vi "Read P T.vi"(1 "correção NTC":dbl, 7 "correçao termopar":dbl) -> (0 "String":string, 2 "Sievert01":dbl, 3 "mean H2 sensor":dbl format="%#_4p", 4 "String 2":string, 5 "mean value T":dbl, 6 "mean value P":dbl, 9 "T Set 1 Output":dbl format="%.4g", 10 "P Set 1 Output 2":dbl format="%.3g", 11 "T Set 2 Output":dbl format="%.4g", 12 "termopar K":dbl format="%.3g", 14 "output NTC":dbl, 15 "P Set 2 Output 2":dbl format="%.3g")   [LabVIEW 2011]
uses:
  <vilib>/Analysis/3filter.llb/Filter Passband Type.ctl
  <vilib>/DAQmx/read.llb/DAQmx Read (Analog 1D DBL 1Chan NSamp).vi
  <vilib>/DAQmx/create/channels.llb/DAQmx Create Channel (AI-Voltage-Basic).vi
  <vilib>/DAQmx/configure/timing.llb/DAQmx Timing (Sample Clock).vi
  <vilib>/DAQmx/miscellaneous.llb/DAQmx Fill In Error Info.vi
  <vilib>/Analysis/3filter.llb/Butterworth Filter (DBL).vi
  <vilib>/Analysis/baseanly.llb/Unimode.vi
  <vilib>/Analysis/5stat.llb/RMS (DBL).vi
  <vilib>/DAQmx/create/channels.llb/DAQmx Create Channel (AI-Temperature-Thermocouple).vi
  <vilib>/Analysis/NI_AALBase.lvlib
  Program Files/National Instruments/LabVIEW 2011/resource/objmgr/daqmx.rc
  <vilib>/gmath/NI_Gmath.lvlib
  <vilib>/Analysis/NI_AALPro.lvlib
panel:
  out "error 4":dbl
  in  "filter type 4":T1
  in  "high cutoff freq: fh 4":dbl=0.45000000000000007 format="%0.2f"
  in  "low cutoff freq: fl 4":dbl=0.12500000000000006 format="%0.4f"
  in  "order 4":i32=2
  in  "intervals 4":i32=20
  out "Rt":dbl
  in  "intervals 3":i32=20
  in  "Statistic 3":T2(ring)
  out "P Set 1 Output 3":dbl format="%.3g"
  out "?":T3(graph)
  out "Data Set 6":dbl[](graph)
  out "?":T3(graph)
  out "Data Set 5":dbl[](graph)
  out "error 3":dbl
  in  "filter type 3":T1
  in  "high cutoff freq: fh 3":dbl=0.45000000000000007 format="%0.2f"
  in  "low cutoff freq: fl 3":dbl=0.12500000000000006 format="%0.4f"
  in  "order 3":i32=2
  out "mean value P 2":dbl
  out "String 3":string
  in  "intervals 2":i32=20
  in  "Statistic 2":T2(ring)
  out "?":T3(graph)
  out "Data Set 4":dbl[](graph)
  out "?":T3(graph)
  out "Data Set 3":dbl[](graph)
  out "error 2":dbl
  in  "filter type 2":T1
  in  "high cutoff freq: fh 2":dbl=0.45000000000000007 format="%0.2f"
  in  "low cutoff freq: fl 2":dbl=0.12500000000000006 format="%0.4f"
  in  "order 2":i32=2
  in  "intervals":i32=20
  in  "Statistic":T2(ring)
  out "?":T3(graph)
  out "Data Set 1":dbl[](graph)
  out "?":T3(graph)
  out "Data Set 2":dbl[](graph)
  out "error":dbl
  in  "filter type":T1
  in  "high cutoff freq: fh":dbl=0.45000000000000007 format="%0.2f"
  in  "low cutoff freq: fl":dbl=0.12500000000000006 format="%0.4f"
  in  "order":i32=2
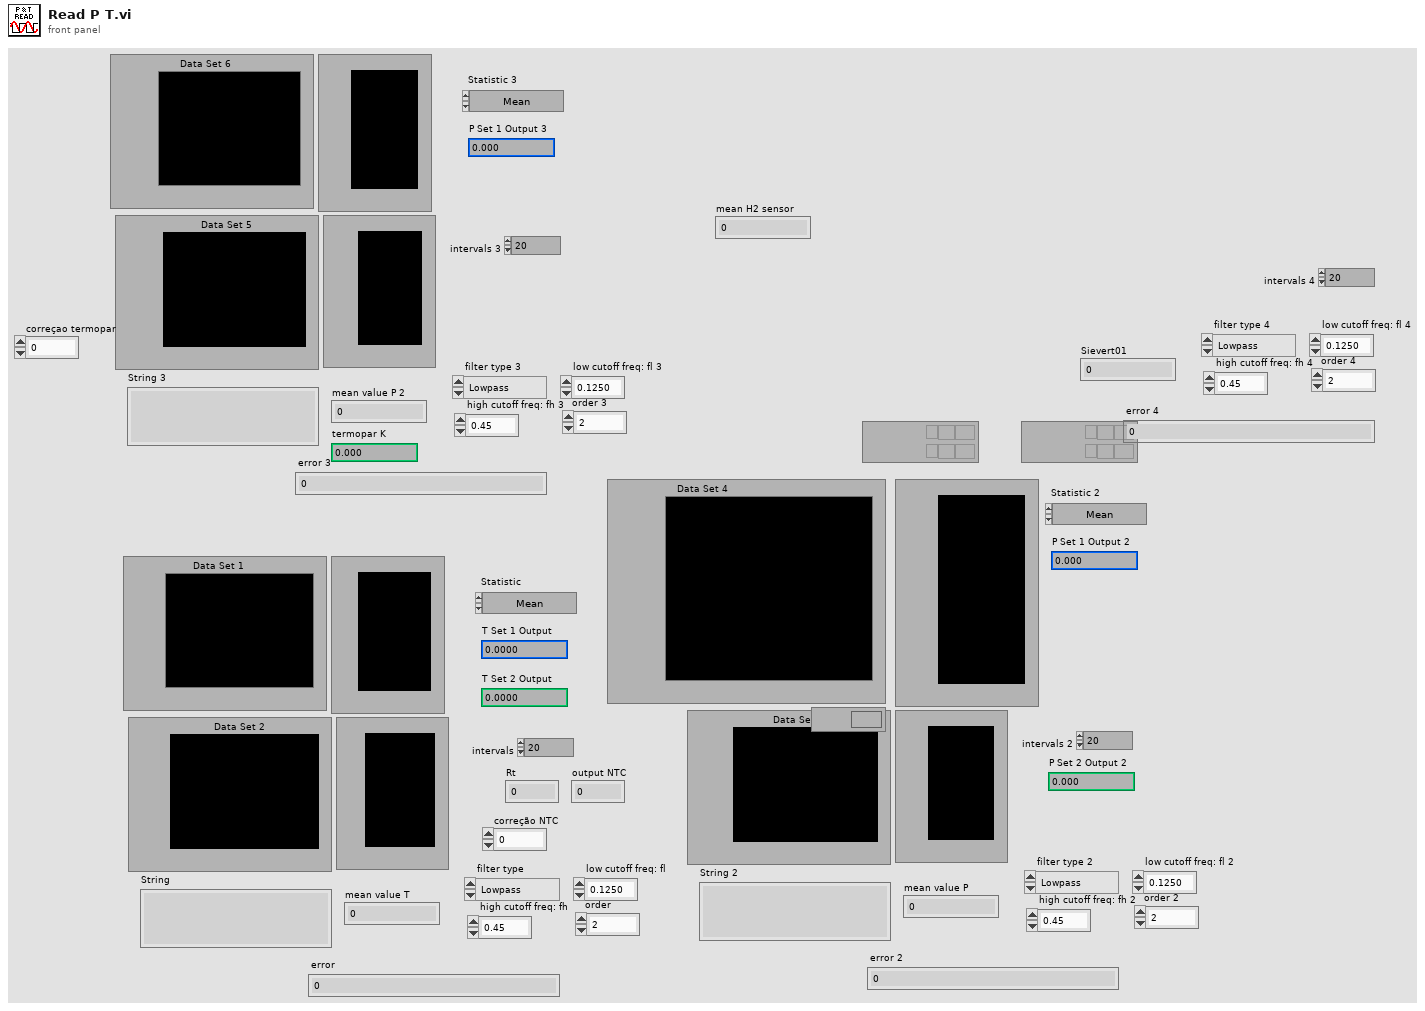
[diagram p1: front panel]
types:
  T1 = typedef "NI_AALBase.lvlib/Filter Passband Type.ctl" = enum32{"Lowpass", "Highpass", "Bandpass", "Bandstop"}
  T2 = enum16{"Mean", "Standard Deviation", "Variance", "Skewness", "Kurtosis", "Median", "Mode", "RMS"}
  T3 = cluster{"Histogram: h(x)":i32[], "X Values":dbl[]}
  T4 = enum16{"arithmetic", "geometric", "harmonic", "trimmed", "median"}
  T5 = cluster{"intervals":i32, "Statistic":enum16{"Mean", "Standard Deviation", "Variance", "Skewness", "Kurtosis", "Median", "Mode", "RMS"}}
  T6 = cluster{"intervals 2":i32, "Statistic 2":enum16{"Mean", "Standard Deviation", "Variance", "Skewness", "Kurtosis", "Median", "Mode", "RMS"}}
  T7 = cluster{"intervals 4":i32, "Statistic 4":enum16{"Mean", "Standard Deviation", "Variance", "Skewness", "Kurtosis", "Median", "Mode", "RMS"}}
  T8 = cluster{"intervals 3":i32, "Statistic 3":enum16{"Mean", "Standard Deviation", "Variance", "Skewness", "Kurtosis", "Median", "Mode", "RMS"}}
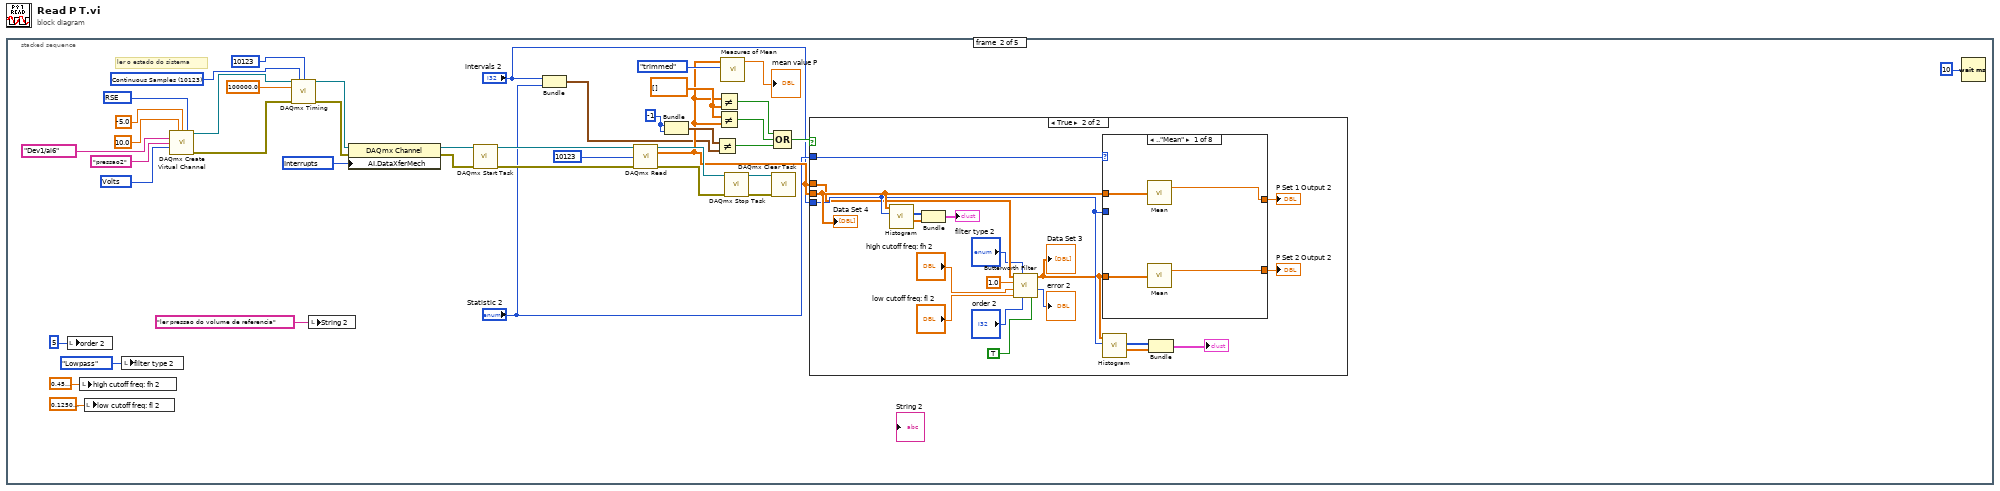
[diagram p0: block diagram]
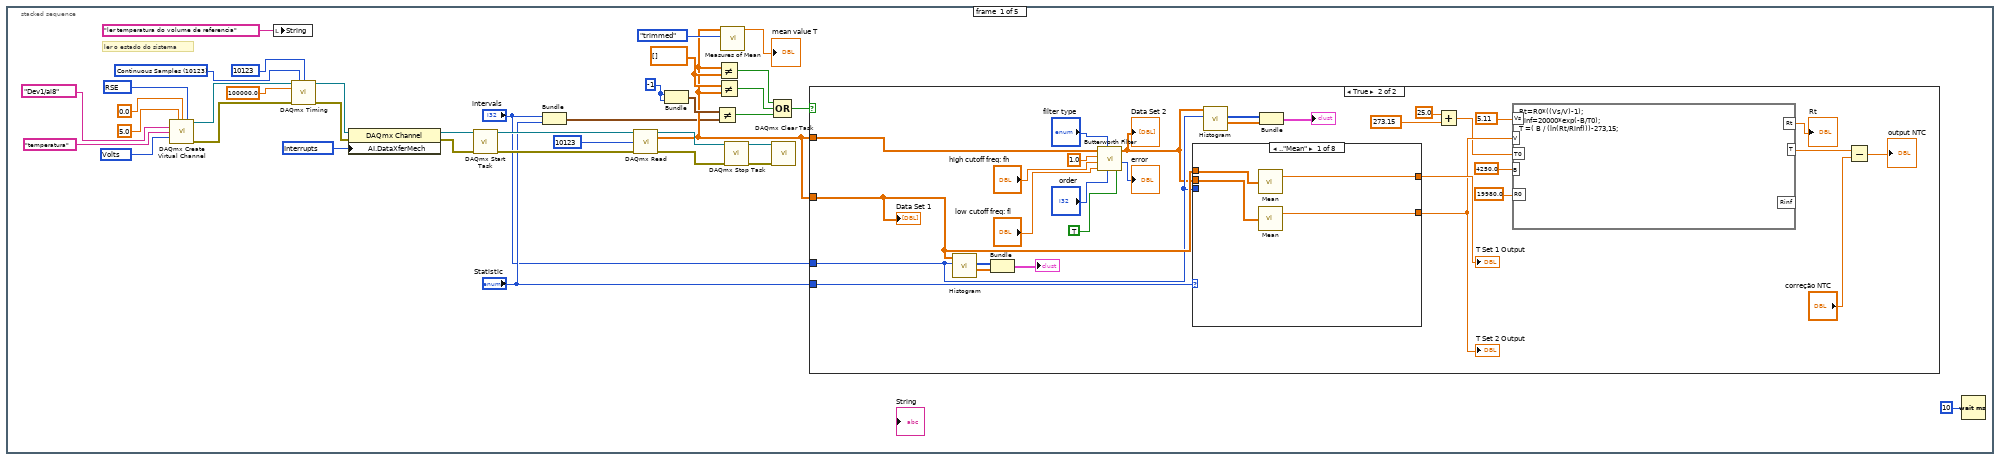
[diagram p2: hidden frame]
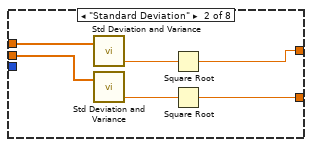
[diagram p4: hidden frame]
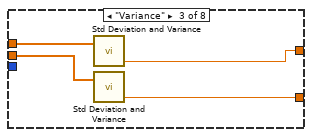
[diagram p5: hidden frame]
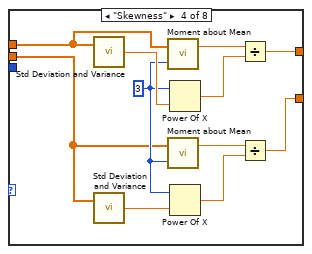
[diagram p6: hidden frame]
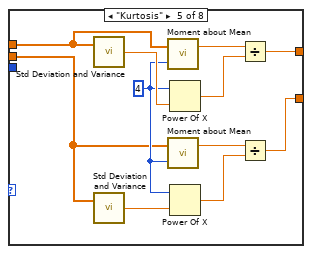
[diagram p7: hidden frame]
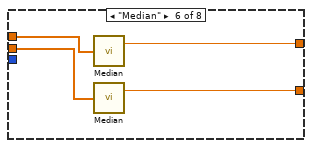
[diagram p8: hidden frame]
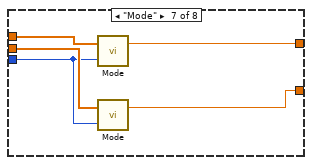
[diagram p9: hidden frame]
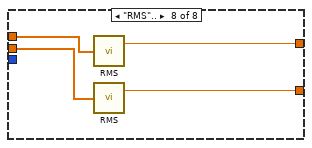
[diagram p10: hidden frame]
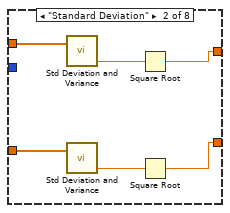
[diagram p12: hidden frame]
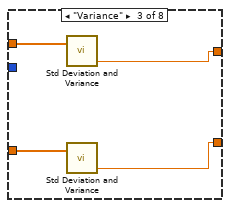
[diagram p13: hidden frame]
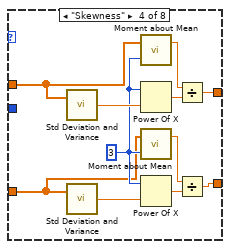
[diagram p14: hidden frame]
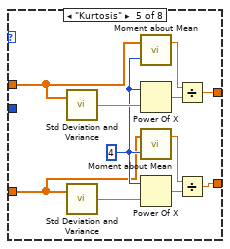
[diagram p15: hidden frame]
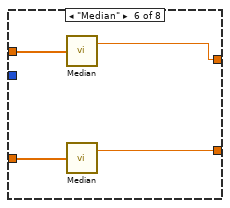
[diagram p16: hidden frame]
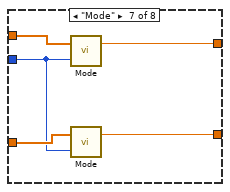
[diagram p17: hidden frame]
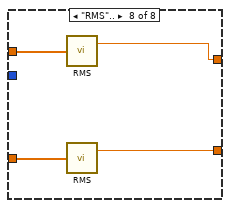
[diagram p18: hidden frame]
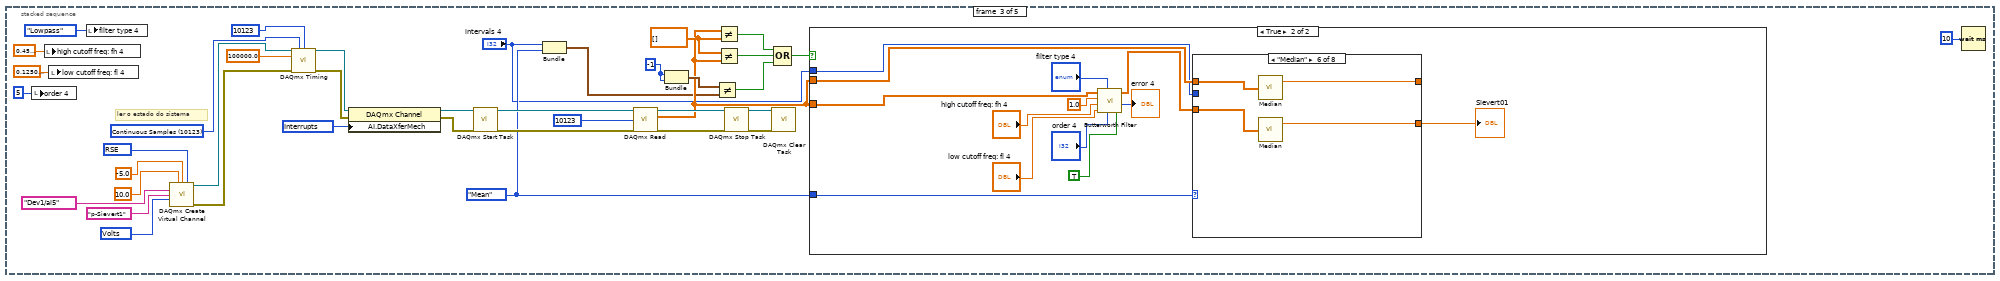
[diagram p19: hidden frame]
diagram:
  n1 = stacked-sequence {
    frame #0 {
      w34 = 10083 items=["default"=-1, "RSE"=10083, "NRSE"=10078, "Differential"=10106, "Pseudodifferential"=12529] ("input terminal configuration")
      w11 = dbl[] []
      w9 = -1
      w27 = 10204 items=["DMA"=10054, "Interrupts"=10204, "Programmed I/O"=10264, "USB Bulk"=12590] ("AI.DataXferMech")
      w30 = 10123 items=["Finite Samples"=10178, "Continuous Samples"=10123, "Hardware Timed Single Point"=12522] ("sample mode")
      w35 = 10348 items=["Volts"=10348, "From Custom Scale"=10065] ("units")
      # "ler o estado do sistema"
      n2 = call-poly <vilib>:"DAQmx Create Virtual Channel.vi"("maximum value"=5.0, "minimum value"=0.0, "input terminal configuration"=w34, "physical channels"=tag "Dev1/ai8" ("P S1"), "name to assign"="temperatura", "units"=w35) -> ("task out"=w24:refnum<k21>, "error out"=w23:errorcluster)  [unwired: 8 in]
      n3 = local write "String"("ler temperatura do volume de referencia" ("String")) -> ()
      n4 = call-poly <vilib>:"DAQmx Timing.vi"("task/channels in"=w24, "sample mode"=w30, "samples per channel"=10123, "rate"=100000.0, "error in"=w23) -> ("task out"=w29:refnum<k21>, "error out"=w28:errorcluster)  [unwired: 9 in]
      n5 = property class="DAQmx Channel"(reference=w29, error in=w28, "AI.DataXferMech"=w27) -> (reference out=w26:refnum<k21>, error out=w25:errorcluster)
      n6 = call <vilib>:"DAQmx Start Task.vi"("task/channels in"=w26, "error in"=w25) -> ("task out"=w32:refnum<k21>, "error out"=w31:errorcluster)  [unwired: 12 in]
      n7 = Bundle("intervals"="intervals", "Statistic"="Statistic") -> (w3:T5)  [unwired: 1 in]
      n8 = call-poly <vilib>:"DAQmx Read.vi"("task/channels in"=w32, "number of samples per channel"=10123, "error in"=w31) -> ("task out"=w16:refnum<k21>, "data"=w8:dbl[], "error out"=w14:errorcluster)  [unwired: 10 in]
      n9 = Bundle(w9, w9) -> (w10:cluster{i32, i32})  [unwired: 1 in]
      n10 = Not Equal?(x=w10, y=w3) -> (x != y?=w2:bool)
      n11 = Not Equal?(x=w8, y=w11) -> (x != y?=w6:bool)
      n12 = Not Equal?(x=w11, y=w8) -> (x != y?=w5:bool)
      n13 = call <vilib>:"Measures of Mean.vi"("type"=T4."trimmed", "x array"=w8) -> ("mean value"=→"mean value T":dbl)  [unwired: 8 in, 1 out]
      n14 = call <vilib>:"DAQmx Stop Task.vi"("task/channels in"=w16, "error in"=w14) -> ("task out"=w15:refnum<k21>, "error out"=w13:errorcluster)  [unwired: 12 in]
      n15 = call <vilib>:"DAQmx Clear Task.vi"("task in"=w15, "error in"=w13) -> ()  [unwired: 13 in, 1 out]
      n16 = Compound Arithmetic op=OR(w6, w5, w2) -> (w7:bool)
      n17 = case shown="True" w7 {
        tunnel: w8 -> [_ w56]
        tunnel: w8 -> [_ w65]
        tunnel: "Statistic" -> [_ w67]
        tunnel: "intervals" -> [_ w63]
        frame False {
        }
        frame True {
          n18 = call <vilib>:"Histogram.vi"("intervals"=w63, "X"=w65) -> ("X Values"=w61:dbl[], "Histogram: h(x)"=w62:i32[])  [unwired: 6 in, 2 out]
          n19 = Bundle("Histogram: h(x)"=w62, "X Values"=w61) -> (→"?":T3)  [unwired: 1 in]
          n20 = call-poly <vilib>:"Butterworth Filter.vi"("init/cont (init:F)"=TRUE, "order"="order", "filter type"="filter type", "low cutoff freq: fl"="low cutoff freq: fl", "high cutoff freq: fh"="high cutoff freq: fh", "sampling freq: fs"=1.0, "X"=w56) -> ("error"=→"error":i32, "Filtered X"=w55:dbl[])  [unwired: 1 in]
          "Data Set 2" <- w55
          n21 = case shown="..\"Mean\"" w67 {
            tunnel: w55 -> [w72 w77 w81 w88 w99 w108 w113 w117]
            tunnel: [w70 w74 w80 w85 w96 w106 w111 w116] -> w47
            tunnel: [w71 w78 w82 w89 w100 w107 w112 w115] -> w68
            tunnel: w65 -> [w69 w73 w79 w92 w103 w105 w110 w114]
            tunnel: w63 -> [_ _ _ _ _ _ w109 _]
            frame .."Mean" {
              n22 = call <vilib>:"Mean.vi"("X"=w69) -> ("mean"=w71:dbl)  [unwired: 1 out]
              n23 = call <vilib>:"Mean.vi"("X"=w72) -> ("mean"=w70:dbl)  [unwired: 1 out]
            }
            frame "Standard Deviation" {
              n24 = call <vilib>:"Std Deviation and Variance.vi"("X"=w73) -> ("variance"=w76:dbl)  [unwired: 1 in, 2 out]
              n25 = call <vilib>:"Std Deviation and Variance.vi"("X"=w77) -> ("variance"=w75:dbl)  [unwired: 1 in, 2 out]
              n26 = Square Root(x=w76) -> (sqrt(x)=w78:dbl)
              n27 = Square Root(x=w75) -> (sqrt(x)=w74:dbl)
            }
            frame "Variance" {
              n28 = call <vilib>:"Std Deviation and Variance.vi"("X"=w79) -> ("variance"=w82:dbl)  [unwired: 1 in, 2 out]
              n29 = call <vilib>:"Std Deviation and Variance.vi"("X"=w81) -> ("variance"=w80:dbl)  [unwired: 1 in, 2 out]
            }
            frame "Skewness" {
              w90 = 3
              n30 = call <vilib>:"Std Deviation and Variance.vi"("X"=w92) -> ("standard deviation"=w93:dbl)  [unwired: 1 in, 2 out]
              n31 = call <vilib>:"Std Deviation and Variance.vi"("X"=w88) -> ("standard deviation"=w91:dbl)  [unwired: 1 in, 2 out]
              n32 = call <vilib>:"Moment about Mean.vi"("order"=w90, "X"=w92) -> ("moment"=w83:dbl)  [unwired: 1 out]
              n33 = call <vilib>:"Moment about Mean.vi"("order"=w90, "X"=w88) -> ("moment"=w86:dbl)  [unwired: 1 out]
              n34 = Power Of X(1:w93, 2:w90) -> (0:w84:dbl)
              n35 = Power Of X(1:w91, 2:w90) -> (0:w87:dbl)
              n36 = Divide(x=w83, y=w84) -> (x/y=w89:dbl)
              n37 = Divide(x=w86, y=w87) -> (x/y=w85:dbl)
            }
            frame "Kurtosis" {
              w101 = 4
              n38 = call <vilib>:"Std Deviation and Variance.vi"("X"=w103) -> ("standard deviation"=w104:dbl)  [unwired: 1 in, 2 out]
              n39 = call <vilib>:"Std Deviation and Variance.vi"("X"=w99) -> ("standard deviation"=w102:dbl)  [unwired: 1 in, 2 out]
              n40 = call <vilib>:"Moment about Mean.vi"("order"=w101, "X"=w103) -> ("moment"=w95:dbl)  [unwired: 1 out]
              n41 = call <vilib>:"Moment about Mean.vi"("order"=w101, "X"=w99) -> ("moment"=w97:dbl)  [unwired: 1 out]
              n42 = Power Of X(1:w104, 2:w101) -> (0:w94:dbl)
              n43 = Power Of X(1:w102, 2:w101) -> (0:w98:dbl)
              n44 = Divide(x=w95, y=w94) -> (x/y=w100:dbl)
              n45 = Divide(x=w97, y=w98) -> (x/y=w96:dbl)
            }
            frame "Median" {
              n46 = call <vilib>:"Median.vi"("X"=w105) -> ("median"=w107:dbl)  [unwired: 1 out]
              n47 = call <vilib>:"Median.vi"("X"=w108) -> ("median"=w106:dbl)  [unwired: 1 out]
            }
            frame "Mode" {
              n48 = call-poly <vilib>:"Mode.vi"("intervals"=w109, "X"=w110) -> ("mode"=w112:dbl)  [unwired: 1 out]
              n49 = call-poly <vilib>:"Mode.vi"("intervals"=w109, "X"=w113) -> ("mode"=w111:dbl)  [unwired: 1 out]
            }
            frame "RMS".. {
              n50 = call-poly <vilib>:"RMS.vi"("X"=w114) -> ("rms value"=w115:dbl)  [unwired: 1 out]
              n51 = call-poly <vilib>:"RMS.vi"("X"=w117) -> ("rms value"=w116:dbl)  [unwired: 1 out]
            }
          }
          "T Set 1 Output" <- w68
          "T Set 2 Output" <- w47
          n52 = call <vilib>:"Histogram.vi"("intervals"=w63, "X"=w55) -> ("X Values"=w59:dbl[], "Histogram: h(x)"=w60:i32[])  [unwired: 6 in, 2 out]
          n53 = Bundle("Histogram: h(x)"=w60, "X Values"=w59) -> (→"?":T3)  [unwired: 1 in]
          n54 = Add(x=25.0 ("T0 (C)"), y=273.15) -> (x+y=w42:dbl)
          n55 = formula code="Rt=R0*((Vs/V)-1);\nRinf=20000*exp(-B/T0);\nT =( B / (ln(Rt/Rinf)))-273,15;"("Vs"=5.11, "V"=w47, "T0"=w42, "B"=4250.0 ("input B"), "R0"=19980.0) -> ("Rt"=→"Rt":dbl, "T"=w40:dbl)  [unwired: 1 out]
          n56 = Subtract(x=w40, y="correção NTC") -> (x-y=→"output NTC":dbl)
          "Data Set 1" <- w65
        }
      }
      n57 = Wait (ms)(milliseconds to wait=u32 10) -> ()  [unwired: 1 out]
    }
    frame #1 {
      w133 = dbl[] []
      w131 = -1
      w150 = 10204 items=["DMA"=10054, "Interrupts"=10204, "Programmed I/O"=10264, "USB Bulk"=12590] ("AI.DataXferMech")
      w153 = 10123 items=["Finite Samples"=10178, "Continuous Samples"=10123, "Hardware Timed Single Point"=12522] ("sample mode")
      w157 = 10083 items=["default"=-1, "RSE"=10083, "NRSE"=10078, "Differential"=10106, "Pseudodifferential"=12529] ("input terminal configuration")
      w158 = 10348 items=["Volts"=10348, "From Custom Scale"=10065] ("units")
      # "ler o estado do sistema"
      n58 = local write "order 2"(5 ("order")) -> ()
      n59 = local write "high cutoff freq: fh 2"(0.45000000000000007 ("high cutoff freq: fh")) -> ()
      n60 = local write "low cutoff freq: fl 2"(0.12500000000000006 ("low cutoff freq: fl")) -> ()
      n61 = local write "filter type 2"(Filter_Passband_Type."Lowpass" ("filter type")) -> ()
      n62 = call-poly <vilib>:"DAQmx Create Virtual Channel.vi"("maximum value"=10.0, "minimum value"=-5.0, "input terminal configuration"=w157, "physical channels"=tag "Dev1/ai6" ("P S1"), "name to assign"="pressao2", "units"=w158) -> ("task out"=w147:refnum<k21>, "error out"=w146:errorcluster)  [unwired: 8 in]
      n63 = call-poly <vilib>:"DAQmx Timing.vi"("task/channels in"=w147, "sample mode"=w153, "samples per channel"=10123, "rate"=100000.0, "error in"=w146) -> ("task out"=w152:refnum<k21>, "error out"=w151:errorcluster)  [unwired: 9 in]
      n64 = local write "String 2"("ler pressao do volume de referencia" ("String")) -> ()
      n65 = property class="DAQmx Channel"(reference=w152, error in=w151, "AI.DataXferMech"=w150) -> (reference out=w149:refnum<k21>, error out=w148:errorcluster)
      n66 = call <vilib>:"DAQmx Start Task.vi"("task/channels in"=w149, "error in"=w148) -> ("task out"=w155:refnum<k21>, "error out"=w154:errorcluster)  [unwired: 12 in]
      n67 = Bundle("intervals 2"="intervals 2", "Statistic 2"="Statistic 2") -> (w125:T6)  [unwired: 1 in]
      n68 = call-poly <vilib>:"DAQmx Read.vi"("task/channels in"=w155, "number of samples per channel"=10123, "error in"=w154) -> ("task out"=w139:refnum<k21>, "data"=w130:dbl[], "error out"=w137:errorcluster)  [unwired: 10 in]
      n69 = Bundle(w131, w131) -> (w132:cluster{i32, i32})  [unwired: 1 in]
      n70 = Not Equal?(x=w132, y=w125) -> (x != y?=w124:bool)
      n71 = Not Equal?(x=w130, y=w133) -> (x != y?=w128:bool)
      n72 = Not Equal?(x=w133, y=w130) -> (x != y?=w127:bool)
      n73 = call <vilib>:"Measures of Mean.vi"("type"=T4."trimmed", "x array"=w130) -> ("mean value"=→"mean value P":dbl)  [unwired: 8 in, 1 out]
      n74 = call <vilib>:"DAQmx Stop Task.vi"("task/channels in"=w139, "error in"=w137) -> ("task out"=w138:refnum<k21>, "error out"=w136:errorcluster)  [unwired: 12 in]
      n75 = call <vilib>:"DAQmx Clear Task.vi"("task in"=w138, "error in"=w136) -> ()  [unwired: 13 in, 1 out]
      n76 = Compound Arithmetic op=OR(w128, w127, w124) -> (w129:bool)
      n77 = case shown="True" w129 {
        tunnel: w130 -> [_ w166]
        tunnel: w130 -> [_ w175]
        tunnel: "Statistic 2" -> [_ w177]
        tunnel: "intervals 2" -> [_ w173]
        frame False {
        }
        frame True {
          n78 = call <vilib>:"Histogram.vi"("intervals"=w173, "X"=w175) -> ("X Values"=w171:dbl[], "Histogram: h(x)"=w172:i32[])  [unwired: 6 in, 2 out]
          n79 = Bundle("Histogram: h(x)"=w172, "X Values"=w171) -> (→"?":T3)  [unwired: 1 in]
          n80 = call-poly <vilib>:"Butterworth Filter.vi"("init/cont (init:F)"=TRUE, "order"="order 2", "filter type"="filter type 2", "low cutoff freq: fl"="low cutoff freq: fl 2", "high cutoff freq: fh"="high cutoff freq: fh 2", "sampling freq: fs"=1.0, "X"=w166) -> ("error"=→"error 2":i32, "Filtered X"=w165:dbl[])  [unwired: 1 in]
          "Data Set 3" <- w165
          n81 = case shown="..\"Mean\"" w177 {
            tunnel: w165 -> [w183 w188 w192 w199 w210 w219 w224 w228]
            tunnel: [w181 w185 w191 w196 w207 w217 w222 w227] -> w178
            tunnel: [w182 w189 w193 w200 w211 w218 w223 w226] -> w179
            tunnel: w175 -> [w180 w184 w190 w203 w214 w216 w221 w225]
            tunnel: w173 -> [_ _ _ _ _ _ w220 _]
            frame .."Mean" {
              n82 = call <vilib>:"Mean.vi"("X"=w180) -> ("mean"=w182:dbl)  [unwired: 1 out]
              n83 = call <vilib>:"Mean.vi"("X"=w183) -> ("mean"=w181:dbl)  [unwired: 1 out]
            }
            frame "Standard Deviation" {
              n84 = call <vilib>:"Std Deviation and Variance.vi"("X"=w184) -> ("variance"=w187:dbl)  [unwired: 1 in, 2 out]
              n85 = call <vilib>:"Std Deviation and Variance.vi"("X"=w188) -> ("variance"=w186:dbl)  [unwired: 1 in, 2 out]
              n86 = Square Root(x=w187) -> (sqrt(x)=w189:dbl)
              n87 = Square Root(x=w186) -> (sqrt(x)=w185:dbl)
            }
            frame "Variance" {
              n88 = call <vilib>:"Std Deviation and Variance.vi"("X"=w190) -> ("variance"=w193:dbl)  [unwired: 1 in, 2 out]
              n89 = call <vilib>:"Std Deviation and Variance.vi"("X"=w192) -> ("variance"=w191:dbl)  [unwired: 1 in, 2 out]
            }
            frame "Skewness" {
              w201 = 3
              n90 = call <vilib>:"Std Deviation and Variance.vi"("X"=w203) -> ("standard deviation"=w204:dbl)  [unwired: 1 in, 2 out]
              n91 = call <vilib>:"Std Deviation and Variance.vi"("X"=w199) -> ("standard deviation"=w202:dbl)  [unwired: 1 in, 2 out]
              n92 = call <vilib>:"Moment about Mean.vi"("order"=w201, "X"=w203) -> ("moment"=w194:dbl)  [unwired: 1 out]
              n93 = Power Of X(1:w204, 2:w201) -> (0:w195:dbl)
              n94 = call <vilib>:"Moment about Mean.vi"("order"=w201, "X"=w199) -> ("moment"=w197:dbl)  [unwired: 1 out]
              n95 = Power Of X(1:w202, 2:w201) -> (0:w198:dbl)
              n96 = Divide(x=w194, y=w195) -> (x/y=w200:dbl)
              n97 = Divide(x=w197, y=w198) -> (x/y=w196:dbl)
            }
            frame "Kurtosis" {
              w212 = 4
              n98 = call <vilib>:"Std Deviation and Variance.vi"("X"=w214) -> ("standard deviation"=w215:dbl)  [unwired: 1 in, 2 out]
              n99 = call <vilib>:"Std Deviation and Variance.vi"("X"=w210) -> ("standard deviation"=w213:dbl)  [unwired: 1 in, 2 out]
              n100 = call <vilib>:"Moment about Mean.vi"("order"=w212, "X"=w214) -> ("moment"=w206:dbl)  [unwired: 1 out]
              n101 = Power Of X(1:w215, 2:w212) -> (0:w205:dbl)
              n102 = call <vilib>:"Moment about Mean.vi"("order"=w212, "X"=w210) -> ("moment"=w208:dbl)  [unwired: 1 out]
              n103 = Power Of X(1:w213, 2:w212) -> (0:w209:dbl)
              n104 = Divide(x=w206, y=w205) -> (x/y=w211:dbl)
              n105 = Divide(x=w208, y=w209) -> (x/y=w207:dbl)
            }
            frame "Median" {
              n106 = call <vilib>:"Median.vi"("X"=w216) -> ("median"=w218:dbl)  [unwired: 1 out]
              n107 = call <vilib>:"Median.vi"("X"=w219) -> ("median"=w217:dbl)  [unwired: 1 out]
            }
            frame "Mode" {
              n108 = call-poly <vilib>:"Mode.vi"("intervals"=w220, "X"=w221) -> ("mode"=w223:dbl)  [unwired: 1 out]
              n109 = call-poly <vilib>:"Mode.vi"("intervals"=w220, "X"=w224) -> ("mode"=w222:dbl)  [unwired: 1 out]
            }
            frame "RMS".. {
              n110 = call-poly <vilib>:"RMS.vi"("X"=w225) -> ("rms value"=w226:dbl)  [unwired: 1 out]
              n111 = call-poly <vilib>:"RMS.vi"("X"=w228) -> ("rms value"=w227:dbl)  [unwired: 1 out]
            }
          }
          "P Set 1 Output 2" <- w179
          "P Set 2 Output 2" <- w178
          n112 = call <vilib>:"Histogram.vi"("intervals"=w173, "X"=w165) -> ("X Values"=w169:dbl[], "Histogram: h(x)"=w170:i32[])  [unwired: 6 in, 2 out]
          n113 = Bundle("Histogram: h(x)"=w170, "X Values"=w169) -> (→"?":T3)  [unwired: 1 in]
          "Data Set 4" <- w175
        }
      }
      n114 = Wait (ms)(milliseconds to wait=u32 10) -> ()  [unwired: 1 out]
    }
    frame #2 {
      w239 = T2."Mean" ("Statistic 4")
      w246 = dbl[] []
      w244 = -1
      w258 = 10204 items=["DMA"=10054, "Interrupts"=10204, "Programmed I/O"=10264, "USB Bulk"=12590] ("AI.DataXferMech")
      w261 = 10123 items=["Finite Samples"=10178, "Continuous Samples"=10123, "Hardware Timed Single Point"=12522] ("sample mode")
      w265 = 10083 items=["default"=-1, "RSE"=10083, "NRSE"=10078, "Differential"=10106, "Pseudodifferential"=12529] ("input terminal configuration")
      w266 = 10348 items=["Volts"=10348, "From Custom Scale"=10065] ("units")
      # "ler o estado do sistema"
      n115 = local write "order 4"(5 ("order")) -> ()
      n116 = local write "high cutoff freq: fh 4"(0.45000000000000007 ("high cutoff freq: fh")) -> ()
      n117 = local write "low cutoff freq: fl 4"(0.12500000000000006 ("low cutoff freq: fl")) -> ()
      n118 = local write "filter type 4"(Filter_Passband_Type."Lowpass" ("filter type")) -> ()
      n119 = call-poly <vilib>:"DAQmx Create Virtual Channel.vi"("maximum value"=10.0, "minimum value"=-5.0, "input terminal configuration"=w265, "physical channels"=tag "Dev1/ai5" ("P S1"), "name to assign"="p-Sievert1", "units"=w266) -> ("task out"=w255:refnum<k21>, "error out"=w254:errorcluster)  [unwired: 8 in]
      n120 = call-poly <vilib>:"DAQmx Timing.vi"("task/channels in"=w255, "sample mode"=w261, "samples per channel"=10123, "rate"=100000.0, "error in"=w254) -> ("task out"=w260:refnum<k21>, "error out"=w259:errorcluster)  [unwired: 9 in]
      n121 = property class="DAQmx Channel"(reference=w260, error in=w259, "AI.DataXferMech"=w258) -> (reference out=w257:refnum<k21>, error out=w256:errorcluster)
      n122 = call <vilib>:"DAQmx Start Task.vi"("task/channels in"=w257, "error in"=w256) -> ("task out"=w263:refnum<k21>, "error out"=w262:errorcluster)  [unwired: 12 in]
      n123 = Bundle("intervals 4"="intervals 4", "Statistic 4"=w239) -> (w238:T7)  [unwired: 1 in]
      n124 = call-poly <vilib>:"DAQmx Read.vi"("task/channels in"=w263, "number of samples per channel"=10123 ("samples per channel"), "error in"=w262) -> ("task out"=w250:refnum<k21>, "data"=w243:dbl[], "error out"=w248:errorcluster)  [unwired: 10 in]
      n125 = Bundle(w244, w244) -> (w245:cluster{i32, i32})  [unwired: 1 in]
      n126 = Not Equal?(x=w245, y=w238) -> (x != y?=w237:bool)
      n127 = Not Equal?(x=w243, y=w246) -> (x != y?=w241:bool)
      n128 = Not Equal?(x=w246, y=w243) -> (x != y?=w240:bool)
      n129 = call <vilib>:"DAQmx Stop Task.vi"("task/channels in"=w250, "error in"=w248) -> ("task out"=w249:refnum<k21>, "error out"=w247:errorcluster)  [unwired: 12 in]
      n130 = call <vilib>:"DAQmx Clear Task.vi"("task in"=w249, "error in"=w247) -> ()  [unwired: 13 in, 1 out]
      n131 = Compound Arithmetic op=OR(w241, w240, w237) -> (w242:bool)
      n132 = case shown="True" w242 {
        tunnel: w243 -> [_ w275]
        tunnel: w243 -> [_ w279]
        tunnel: w239 -> [_ w280]
        tunnel: "intervals 4" -> [_ w278]
        frame False {
        }
        frame True {
          n133 = call-poly <vilib>:"Butterworth Filter.vi"("init/cont (init:F)"=TRUE, "order"="order 4", "filter type"="filter type 4", "low cutoff freq: fl"="low cutoff freq: fl 4", "high cutoff freq: fh"="high cutoff freq: fh 4", "sampling freq: fs"=1.0, "X"=w275) -> ("error"=→"error 4":i32, "Filtered X"=w274:dbl[])  [unwired: 1 in]
          n134 = case shown="\"Median\"" w280 {
            tunnel: w274 -> [w284 w289 w293 w300 w311 w320 w325 w329]
            tunnel: [w282 w286 w292 w297 w308 w318 w323 w328] -> w268
            tunnel: [w283 w290 w294 w301 w312 w319 w324 w327] -> _
            tunnel: w279 -> [w281 w285 w291 w304 w315 w317 w322 w326]
            tunnel: w278 -> [_ _ _ _ _ _ w321 _]
            frame .."Mean" {
              n135 = call <vilib>:"Mean.vi"("X"=w281) -> ("mean"=w283:dbl)  [unwired: 1 out]
              n136 = call <vilib>:"Mean.vi"("X"=w284) -> ("mean"=w282:dbl)  [unwired: 1 out]
            }
            frame "Standard Deviation" {
              n137 = call <vilib>:"Std Deviation and Variance.vi"("X"=w285) -> ("variance"=w288:dbl)  [unwired: 1 in, 2 out]
              n138 = call <vilib>:"Std Deviation and Variance.vi"("X"=w289) -> ("variance"=w287:dbl)  [unwired: 1 in, 2 out]
              n139 = Square Root(x=w288) -> (sqrt(x)=w290:dbl)
              n140 = Square Root(x=w287) -> (sqrt(x)=w286:dbl)
            }
            frame "Variance" {
              n141 = call <vilib>:"Std Deviation and Variance.vi"("X"=w291) -> ("variance"=w294:dbl)  [unwired: 1 in, 2 out]
              n142 = call <vilib>:"Std Deviation and Variance.vi"("X"=w293) -> ("variance"=w292:dbl)  [unwired: 1 in, 2 out]
            }
            frame "Skewness" {
              w302 = 3
              n143 = call <vilib>:"Std Deviation and Variance.vi"("X"=w304) -> ("standard deviation"=w305:dbl)  [unwired: 1 in, 2 out]
              n144 = call <vilib>:"Std Deviation and Variance.vi"("X"=w300) -> ("standard deviation"=w303:dbl)  [unwired: 1 in, 2 out]
              n145 = call <vilib>:"Moment about Mean.vi"("order"=w302, "X"=w304) -> ("moment"=w295:dbl)  [unwired: 1 out]
              n146 = call <vilib>:"Moment about Mean.vi"("order"=w302, "X"=w300) -> ("moment"=w298:dbl)  [unwired: 1 out]
              n147 = Power Of X(1:w305, 2:w302) -> (0:w296:dbl)
              n148 = Power Of X(1:w303, 2:w302) -> (0:w299:dbl)
              n149 = Divide(x=w295, y=w296) -> (x/y=w301:dbl)
              n150 = Divide(x=w298, y=w299) -> (x/y=w297:dbl)
            }
            frame "Kurtosis" {
              w313 = 4
              n151 = call <vilib>:"Std Deviation and Variance.vi"("X"=w315) -> ("standard deviation"=w316:dbl)  [unwired: 1 in, 2 out]
              n152 = call <vilib>:"Std Deviation and Variance.vi"("X"=w311) -> ("standard deviation"=w314:dbl)  [unwired: 1 in, 2 out]
              n153 = call <vilib>:"Moment about Mean.vi"("order"=w313, "X"=w315) -> ("moment"=w307:dbl)  [unwired: 1 out]
              n154 = call <vilib>:"Moment about Mean.vi"("order"=w313, "X"=w311) -> ("moment"=w309:dbl)  [unwired: 1 out]
              n155 = Power Of X(1:w316, 2:w313) -> (0:w306:dbl)
              n156 = Power Of X(1:w314, 2:w313) -> (0:w310:dbl)
              n157 = Divide(x=w307, y=w306) -> (x/y=w312:dbl)
              n158 = Divide(x=w309, y=w310) -> (x/y=w308:dbl)
            }
            frame "Median" {
              n159 = call <vilib>:"Median.vi"("X"=w317) -> ("median"=w319:dbl)  [unwired: 1 out]
              n160 = call <vilib>:"Median.vi"("X"=w320) -> ("median"=w318:dbl)  [unwired: 1 out]
            }
            frame "Mode" {
              n161 = call-poly <vilib>:"Mode.vi"("intervals"=w321, "X"=w322) -> ("mode"=w324:dbl)  [unwired: 1 out]
              n162 = call-poly <vilib>:"Mode.vi"("intervals"=w321, "X"=w325) -> ("mode"=w323:dbl)  [unwired: 1 out]
            }
            frame "RMS".. {
              n163 = call-poly <vilib>:"RMS.vi"("X"=w326) -> ("rms value"=w327:dbl)  [unwired: 1 out]
              n164 = call-poly <vilib>:"RMS.vi"("X"=w329) -> ("rms value"=w328:dbl)  [unwired: 1 out]
            }
          }
          "Sievert01" <- w268
        }
      }
      n165 = Wait (ms)(milliseconds to wait=u32 10) -> ()  [unwired: 1 out]
    }
    frame #3 {
      w347 = 10204 items=["DMA"=10054, "Interrupts"=10204, "Programmed I/O"=10264, "USB Bulk"=12590] ("AI.DataXferMech")
      w350 = 10123 items=["Finite Samples"=10178, "Continuous Samples"=10123, "Hardware Timed Single Point"=12522] ("sample mode")
      w354 = 10106 items=["default"=-1, "RSE"=10083, "NRSE"=10078, "Differential"=10106, "Pseudodifferential"=12529] ("input terminal configuration")
      w355 = 10348 items=["Volts"=10348, "From Custom Scale"=10065] ("units")
      # "ler o estado do sistema"
      n166 = call-poly <vilib>:"DAQmx Create Virtual Channel.vi"("maximum value"=5.0, "minimum value"=0.0, "input terminal configuration"=w354, "physical channels"=tag "Dev1/ai1" ("P S1"), "name to assign"="H2 sensor", "units"=w355) -> ("task out"=w344:refnum<k21>, "error out"=w343:errorcluster)  [unwired: 8 in]
      n167 = call-poly <vilib>:"DAQmx Timing.vi"("task/channels in"=w344, "sample mode"=w350, "samples per channel"=10123, "rate"=100000.0, "error in"=w343) -> ("task out"=w349:refnum<k21>, "error out"=w348:errorcluster)  [unwired: 9 in]
      n168 = property class="DAQmx Channel"(reference=w349, error in=w348, "AI.DataXferMech"=w347) -> (reference out=w346:refnum<k21>, error out=w345:errorcluster)
      n169 = call <vilib>:"DAQmx Start Task.vi"("task/channels in"=w346, "error in"=w345) -> ("task out"=w352:refnum<k21>, "error out"=w351:errorcluster)  [unwired: 12 in]
      n170 = call-poly <vilib>:"DAQmx Read.vi"("task/channels in"=w352, "number of samples per channel"=10123, "error in"=w351) -> ("task out"=w336:refnum<k21>, "data"=w331:dbl[], "error out"=w334:errorcluster)  [unwired: 10 in]
      n171 = call <vilib>:"Measures of Mean.vi"("type"=T4."trimmed", "x array"=w331) -> ("mean value"=→"mean H2 sensor":dbl)  [unwired: 8 in, 1 out]
      n172 = call <vilib>:"DAQmx Stop Task.vi"("task/channels in"=w336, "error in"=w334) -> ("task out"=w335:refnum<k21>, "error out"=w333:errorcluster)  [unwired: 12 in]
      n173 = call <vilib>:"DAQmx Clear Task.vi"("task in"=w335, "error in"=w333) -> ()  [unwired: 13 in, 1 out]
      n174 = Wait (ms)(milliseconds to wait=u32 10) -> ()  [unwired: 1 out]
    }
    frame #4 {
      w360 = 10116 items=["Built-In"=10200, "Constant Value"=10116, "Channel"=10113] ("cjc source")
      w363 = 10073 items=["J"=10072, "K"=10073, "N"=10077, "R"=10082, "S"=10085, "T"=10086, "B"=10047, "E"=10055] ("thermocouple type")
      w364 = 10143 items=["Deg C"=10143, "Deg F"=10144, "Kelvins"=10325, "Deg R"=10145, "From Custom Scale"=10065] ("units")
      w379 = dbl[] []
      w377 = -1
      w394 = 10204 items=["DMA"=10054, "Interrupts"=10204, "Programmed I/O"=10264, "USB Bulk"=12590] ("AI.DataXferMech")
      w397 = 10123 items=["Finite Samples"=10178, "Continuous Samples"=10123, "Hardware Timed Single Point"=12522] ("sample mode")
      # "ler o estado do sistema"
      n175 = local write "order 3"(5 ("order")) -> ()
      n176 = local write "high cutoff freq: fh 3"(0.45000000000000007 ("high cutoff freq: fh")) -> ()
      n177 = local write "low cutoff freq: fl 3"(0.12500000000000006 ("low cutoff freq: fl")) -> ()
      n178 = property on="output NTC" class="DigNum (strict)"() -> ("Value"=w359:dbl)  [unwired: 2 in, 2 out]
      n179 = Add(x=w359, y="correçao termopar") -> (x+y=w358:dbl)
      n180 = local write "String 3"("ler pressao do volume de referencia" ("String")) -> ()
      n181 = call-poly <vilib>:"DAQmx Create Virtual Channel.vi"("maximum value"=500.0, "minimum value"=-200.0, "physical channels"=tag "Dev1/ai15" ("P S1"), "cjc source"=w360, "name to assign"="termopar K", "units"=w364, "thermocouple type"=w363, "cjc value"=w358) -> ("task out"=w391:refnum<k21>, "error out"=w390:errorcluster)  [unwired: 6 in]
      n182 = call-poly <vilib>:"DAQmx Timing.vi"("task/channels in"=w391, "sample mode"=w397, "samples per channel"=1000, "rate"=100000.0, "error in"=w390) -> ("task out"=w396:refnum<k21>, "error out"=w395:errorcluster)  [unwired: 9 in]
      n183 = property class="DAQmx Channel"(reference=w396, error in=w395, "AI.DataXferMech"=w394) -> (reference out=w393:refnum<k21>, error out=w392:errorcluster)
      n184 = call <vilib>:"DAQmx Start Task.vi"("task/channels in"=w393, "error in"=w392) -> ("task out"=w399:refnum<k21>, "error out"=w398:errorcluster)  [unwired: 12 in]
      n185 = Bundle("intervals 3"="intervals 3", "Statistic 3"="Statistic 3") -> (w371:T8)  [unwired: 1 in]
      n186 = call-poly <vilib>:"DAQmx Read.vi"("task/channels in"=w399, "number of samples per channel"=1000, "error in"=w398) -> ("task out"=w385:refnum<k21>, "data"=w376:dbl[], "error out"=w383:errorcluster)  [unwired: 10 in]
      n187 = Bundle(w377, w377) -> (w378:cluster{i32, i32})  [unwired: 1 in]
      n188 = Not Equal?(x=w378, y=w371) -> (x != y?=w370:bool)
      n189 = Not Equal?(x=w376, y=w379) -> (x != y?=w374:bool)
      n190 = Not Equal?(x=w379, y=w376) -> (x != y?=w373:bool)
      n191 = call <vilib>:"Measures of Mean.vi"("type"=T4."trimmed", "x array"=w376) -> ("mean value"=→"mean value P 2":dbl)  [unwired: 8 in, 1 out]
      n192 = call <vilib>:"DAQmx Stop Task.vi"("task/channels in"=w385, "error in"=w383) -> ("task out"=w384:refnum<k21>, "error out"=w382:errorcluster)  [unwired: 12 in]
      n193 = call <vilib>:"DAQmx Clear Task.vi"("task in"=w384, "error in"=w382) -> ()  [unwired: 13 in, 1 out]
      n194 = Compound Arithmetic op=OR(w374, w373, w370) -> (w375:bool)
      n195 = case shown="True" w375 {
        tunnel: w376 -> [_ w411]
        tunnel: w376 -> [_ w420]
        tunnel: "Statistic 3" -> [_ w422]
        tunnel: "intervals 3" -> [_ w418]
        frame False {
        }
        frame True {
          n196 = call <vilib>:"Histogram.vi"("intervals"=w418, "X"=w420) -> ("X Values"=w416:dbl[], "Histogram: h(x)"=w417:i32[])  [unwired: 6 in, 2 out]
          n197 = Bundle("Histogram: h(x)"=w417, "X Values"=w416) -> (→"?":T3)  [unwired: 1 in]
          n198 = call-poly <vilib>:"Butterworth Filter.vi"("init/cont (init:F)"=TRUE, "order"="order 3", "filter type"="filter type 3", "low cutoff freq: fl"="low cutoff freq: fl 3", "high cutoff freq: fh"="high cutoff freq: fh 3", "sampling freq: fs"=1.0, "X"=w411) -> ("error"=→"error 3":i32, "Filtered X"=w410:dbl[])  [unwired: 1 in]
          "Data Set 5" <- w410
          n199 = case shown="\"Median\"" w422 {
            tunnel: w410 -> [w427 w432 w436 w443 w454 w463 w468 w472]
            tunnel: [w425 w429 w435 w440 w451 w461 w466 w471] -> w403
            tunnel: [w426 w433 w437 w444 w455 w462 w467 w470] -> w423
            tunnel: w420 -> [w424 w428 w434 w447 w458 w460 w465 w469]
            tunnel: w418 -> [_ _ _ _ _ _ w464 _]
            frame .."Mean" {
              n200 = call <vilib>:"Mean.vi"("X"=w427) -> ("mean"=w425:dbl)  [unwired: 1 out]
              n201 = call <vilib>:"Mean.vi"("X"=w424) -> ("mean"=w426:dbl)  [unwired: 1 out]
            }
            frame "Standard Deviation" {
              n202 = call <vilib>:"Std Deviation and Variance.vi"("X"=w432) -> ("variance"=w430:dbl)  [unwired: 1 in, 2 out]
              n203 = call <vilib>:"Std Deviation and Variance.vi"("X"=w428) -> ("variance"=w431:dbl)  [unwired: 1 in, 2 out]
              n204 = Square Root(x=w430) -> (sqrt(x)=w429:dbl)
              n205 = Square Root(x=w431) -> (sqrt(x)=w433:dbl)
            }
            frame "Variance" {
              n206 = call <vilib>:"Std Deviation and Variance.vi"("X"=w436) -> ("variance"=w435:dbl)  [unwired: 1 in, 2 out]
              n207 = call <vilib>:"Std Deviation and Variance.vi"("X"=w434) -> ("variance"=w437:dbl)  [unwired: 1 in, 2 out]
            }
            frame "Skewness" {
              w445 = 3
              n208 = call <vilib>:"Std Deviation and Variance.vi"("X"=w443) -> ("standard deviation"=w446:dbl)  [unwired: 1 in, 2 out]
              n209 = call <vilib>:"Std Deviation and Variance.vi"("X"=w447) -> ("standard deviation"=w448:dbl)  [unwired: 1 in, 2 out]
              n210 = call <vilib>:"Moment about Mean.vi"("order"=w445, "X"=w443) -> ("moment"=w441:dbl)  [unwired: 1 out]
              n211 = call <vilib>:"Moment about Mean.vi"("order"=w445, "X"=w447) -> ("moment"=w438:dbl)  [unwired: 1 out]
              n212 = Power Of X(1:w446, 2:w445) -> (0:w442:dbl)
              n213 = Power Of X(1:w448, 2:w445) -> (0:w439:dbl)
              n214 = Divide(x=w441, y=w442) -> (x/y=w440:dbl)
              n215 = Divide(x=w438, y=w439) -> (x/y=w444:dbl)
            }
            frame "Kurtosis" {
              w456 = 4
              n216 = call <vilib>:"Std Deviation and Variance.vi"("X"=w454) -> ("standard deviation"=w457:dbl)  [unwired: 1 in, 2 out]
              n217 = call <vilib>:"Std Deviation and Variance.vi"("X"=w458) -> ("standard deviation"=w459:dbl)  [unwired: 1 in, 2 out]
              n218 = call <vilib>:"Moment about Mean.vi"("order"=w456, "X"=w454) -> ("moment"=w452:dbl)  [unwired: 1 out]
              n219 = call <vilib>:"Moment about Mean.vi"("order"=w456, "X"=w458) -> ("moment"=w450:dbl)  [unwired: 1 out]
              n220 = Power Of X(1:w457, 2:w456) -> (0:w453:dbl)
              n221 = Power Of X(1:w459, 2:w456) -> (0:w449:dbl)
              n222 = Divide(x=w452, y=w453) -> (x/y=w451:dbl)
              n223 = Divide(x=w450, y=w449) -> (x/y=w455:dbl)
            }
            frame "Median" {
              n224 = call <vilib>:"Median.vi"("X"=w463) -> ("median"=w461:dbl)  [unwired: 1 out]
              n225 = call <vilib>:"Median.vi"("X"=w460) -> ("median"=w462:dbl)  [unwired: 1 out]
            }
            frame "Mode" {
              n226 = call-poly <vilib>:"Mode.vi"("intervals"=w464, "X"=w468) -> ("mode"=w466:dbl)  [unwired: 1 out]
              n227 = call-poly <vilib>:"Mode.vi"("intervals"=w464, "X"=w465) -> ("mode"=w467:dbl)  [unwired: 1 out]
            }
            frame "RMS".. {
              n228 = call-poly <vilib>:"RMS.vi"("X"=w472) -> ("rms value"=w471:dbl)  [unwired: 1 out]
              n229 = call-poly <vilib>:"RMS.vi"("X"=w469) -> ("rms value"=w470:dbl)  [unwired: 1 out]
            }
          }
          "P Set 1 Output 3" <- w423
          n230 = call <vilib>:"Histogram.vi"("intervals"=w418, "X"=w410) -> ("X Values"=w414:dbl[], "Histogram: h(x)"=w415:i32[])  [unwired: 6 in, 2 out]
          n231 = Bundle("Histogram: h(x)"=w415, "X Values"=w414) -> (→"?":T3)  [unwired: 1 in]
          n232 = Subtract(x=w403, y=0.0 ("correçao termo k")) -> (x-y=→"termopar K":dbl)
          "Data Set 6" <- w420
        }
      }
      n233 = Wait (ms)(milliseconds to wait=u32 10) -> ()  [unwired: 1 out]
    }
  }
